vi "Set SET parameters.vi"(8 "error in (no error)":errorcluster, 11 "Simulated_CCD_Camera in":refnum<class "Simulated_CCD_Camera.lvclass">) -> (0 "error out":errorcluster, 3 "Simulated_CCD_Camera out":refnum<class "Simulated_CCD_Camera.lvclass">)   [LabVIEW 2018, in "Simulated_CCD_Camera.lvclass"]
uses:
  Simulated_CCD_Camera.lvclass
  Simulated_CCD_Camera.lvclass/Simulated_CCD_Camera.ctl
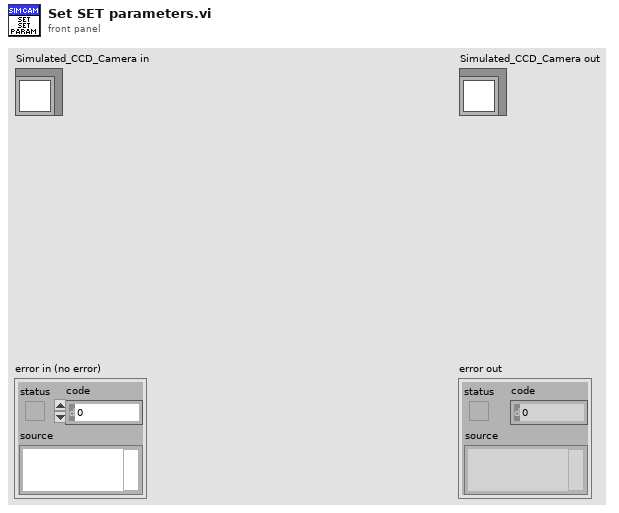
[diagram p1: front panel]
types:
  T1 = cluster{"COOLER_POWER_STATUS":u16, "TEMP":i32, "EXPTIME":dbl, "#FRAMES":u32, "#CYCLES":u32, "#SEQS":u32, "WAVEPLATE_POS":u16}
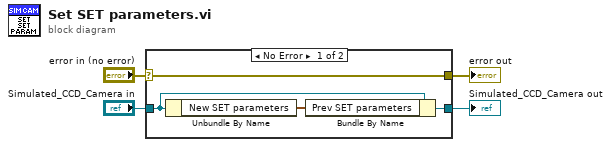
[diagram p0: block diagram]
diagram:
  n1 = case shown="No Error" "error in (no error)" {
    selector: "error in (no error)" -> [w8 w10]
    tunnel: [w8 w10] -> w3
    tunnel: [w6 w9] -> w1
    tunnel: "Simulated_CCD_Camera in" -> [w7 w9]
    frame No Error {
      n2 = Unbundle By Name(w7) -> ("New SET parameters"=w5:T1)
      n3 = Bundle By Name(cluster=w7, "Prev SET parameters"=w5) -> (w6:refnum<class "Simulated_CCD_Camera.lvclass">)
    }
    frame Error {
    }
  }
  "error out" <- w3
  "Simulated_CCD_Camera out" <- w1
